vi "String Compare (case insensitive).vi"(8 "error in (no error)":errorcluster, 9 "string B":string, 10 "string A":string) -> (0 "error out":errorcluster, 2 "result":i32)   [LabVIEW 2014, in "SQLite3LV.lvlib" / "sqlite3.lvclass"]
doc: "String Comparison\n\n int SQLite3LV Connection_stricmp(const char *, const char *);\n int sqlite3_strnicmp(const char *, const char *, int);\n\nThe sqlite3_stricmp() and sqlite3_strnicmp() APIs allow applications and extensions to compare the contents of two buffers containing UTF-8 strings in a case-independent fashion, using the same definition of \"case independence\" that SQLite uses internally when comparing identifiers."
uses:
  sqlite3.lvclass
  sqlite3_64.dll
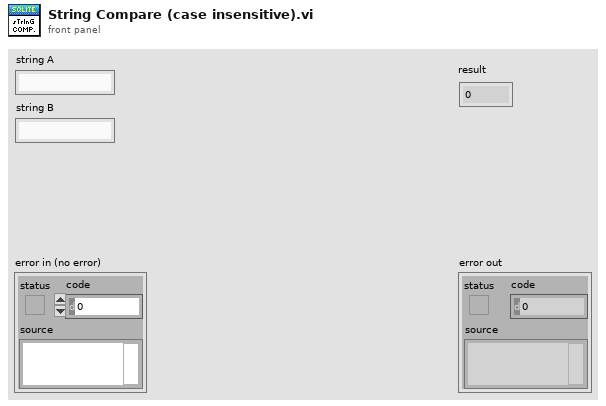
[diagram p1: front panel]
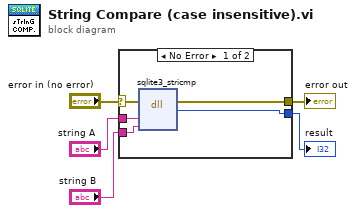
[diagram p0: block diagram]
diagram:
  n1 = case shown="No Error" "error in (no error)" {
    selector: "error in (no error)" -> [w10 w11]
    tunnel: [w9 w11] -> w4
    tunnel: "string A" -> [w7 _]
    tunnel: "string B" -> [w6 _]
    tunnel: [w8 _] -> w1
    frame No Error {
      n2 = dll-call lib="C:/Users/BobUser/Desktop/LVTables/sqlite3**.*" fn="sqlite3_stricmp"(error in=w10, "string A"=w7, "string B"=w6) -> (error out=w9:errorcluster, "result"=w8:i32)  [unwired: 4 in, 1 out]
    }
    frame Error {
    }
  }
  "error out" <- w4
  "result" <- w1
